vi "SV Get By Measurement Type (prox probe) (N Ch).vi"(0 "scaled signals [EU]":waveform(dbl)[](array[waveform])) -> (4 "scaled signals with proximity channels deleted":waveform(dbl)[](array[waveform]), 6 "number of proximity channels":i32, 8 "proximity probe channels":waveform(dbl)[](array[waveform]), 10 "pair":i32[](array[numeric]), 15 "probe angle":dbl[](array[numeric]))   [LabVIEW 2017]
doc: "Separates data from an array of waveforms based on the type of measurement selected. This VI requires that waveform attributes such as NI_UnitDescription are added by NI DAQmx."
uses:
  <vilib>/addons/_NISVFA/_Shared subVIs/Controls/SV Channel Properties.ctl
  <vilib>/addons/_NISVFA/_Shared subVIs/Groups/SV Match Unit.vi
  <vilib>/addons/_NISVFA/_Shared subVIs/Common/sv_Get NI Property Name String.vi
  <vilib>/addons/_NISVFA/_Shared subVIs/Groups/sv_ConcatenateArrayIndicies.vi
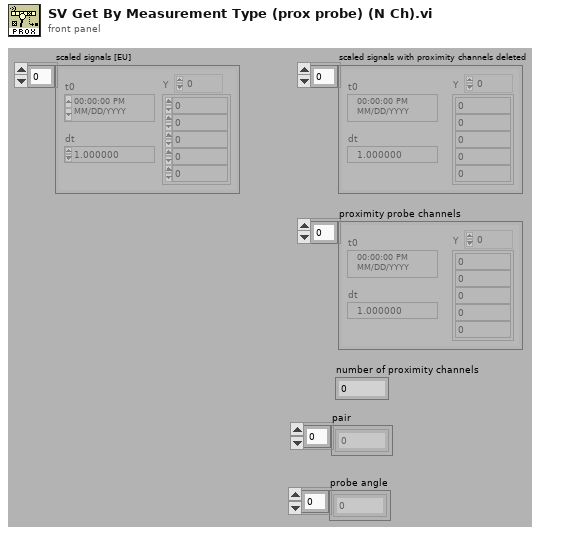
[diagram p1: front panel]
types:
  T1 = typedef "SV Channel Properties.ctl" = u16
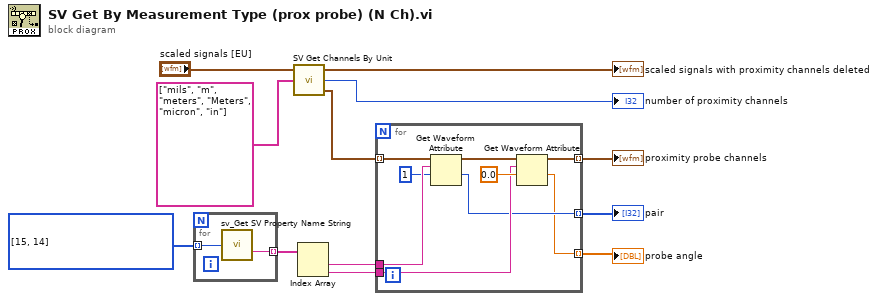
[diagram p0: block diagram]
diagram:
  w6 = T1[] [15, 14] items=["Engineering units", "Custom unit label", "Weighting filter", "Pregain", "Octave standard", "Octave bandwidth", "Octave low band", "Octave high band", "Spectrum skewed", "Samples / revolution", "Order", "Tachometer", "Pulses Per Revolution", "Rotation Direction", "Probe Angle", "Pair", "Channel Alias", "Tachometer Threshold", "Tachometer Slope", "Max Order", "Sensor Location", "Sensor Orientation"]
  n1 = for {
    tunnel: w6 -> [w14] mode=indexing
    tunnel: [w13] -> w5 mode=indexing
    n2 = call <vilib>:"sv_Get SV Property Name String.vi"("property"=w14) -> ("WDT attribute name"=w13:string)  [unwired: 13 in, 1 out]
  }
  n3 = call <vilib>:"SV Get Channels By Unit.vi"("units to match"=string[] ["mils", "m", "meters", "Meters", "micron", "in"] ("Units to Match"), "scaled signals [EU]"="scaled signals [EU]") -> ("matching channels [EU]"=w8:waveform(dbl)[], "number of matching channels"=→"number of proximity channels":i32, "scaled signals with matching channels deleted"=→"scaled signals with proximity channels deleted":waveform(dbl)[])  [unwired: 1 in]
  n4 = Index Array(array=w5) -> (element #1=w4:string, element #2=w3:string)  [unwired: 2 in]
  n5 = for {
    tunnel: w8 -> [w23] mode=indexing
    tunnel: [w19] -> w7 mode=indexing
    tunnel: w4 -> [w22]
    tunnel: w3 -> [w17]
    tunnel: [w16] -> w2 mode=indexing
    tunnel: [w15] -> w1 mode=indexing
    n6 = Get Waveform Attribute(5:1, 6:w22, 7:w23) -> (1:w16:i32, 3:w20:waveform(dbl))  [unwired: 1 in, 2 out]
    n7 = Get Waveform Attribute(5:0.0, 6:w17, 7:w20) -> (1:w15:dbl, 3:w19:waveform(dbl))  [unwired: 1 in, 2 out]
  }
  "proximity probe channels" <- w7
  "pair" <- w2
  "probe angle" <- w1
